vi "FRIC_navX_Internal_I2C_ProcessingLoop.vi"(10 "I2C Bus (in)":T3=enum."Invalid", 11 "Update Rate (4Hz-100Hz)":u8=50 min=4 max=100) -> (0 "error out":errorcluster)   [LabVIEW 2015]
doc: "This navX VI handles the reading/writing for the navX. All of the good stuff is in here.\nTHIS VI SHOULD NOT BE CALLED BY THE USER!"
uses:
  <vilib>/Rock Robotics/SystemInterfaces/i2clib/i2c_bus.ctl
  navX Library v2/_TypeDefs/Z900_navX_DeviceTypeDef.ctl
  navX Library v2/_TypeDefs/Z900_navX_ProtocolTypeDef.ctl
  navX Library v2/_TypeDefs/Z900_navX_NotifyPacketTypeDef.ctl
  navX Library v2/_TypeDefs/Z900_navX_ActionTypeDef.ctl
  TypeDefs/FRIC_navX_ProcessingLoopStatesTypeDef_I2C.ctl
  TypeDefs/FRIC_navX_I2C Process Loop TypeDef.ctl
  <vilib>/Rock Robotics/SystemInterfaces/Typedef/FPGA_TypedefDigitalModule.ctl
  navX Library v2/_TypeDefs/Z900_navX_IntegrationControlRegisters.ctl
  <vilib>/Rock Robotics/WPI/SPI/WPI_SPIDevRef.ctl
  <vilib>/Rock Robotics/SystemInterfaces/spilib/spi_bus.ctl
  _NI WPI Serial USB/WPI_SerialPort_USB.ctl
  navX Library v2/_TypeDefs/Z900_navX_SerialStreamTypeDef.ctl
  <vilib>/Rock Robotics/WPI/SerialPort/WPI_SerialPortRef.ctl
  navX Library v2/_TypeDefs/Flags/Z900_navX_Flags_CapabilityTypeDef.ctl
  navX Library v2/_TypeDefs/Z900_navX_DeviceRegisters.ctl
  navX Library v2/_TypeDefs/navX Open TypeDefs/Z900_navX_OpenTypeDef_I2C.ctl
  <vilib>/Rock Robotics/SystemInterfaces/Utilities/FPGA_UtilitiesRead LocalTime.vi
  navX Library v2/navX Library v2.lvlib
  _NI WPI Serial USB/_NI WPI Serial USB.lvlib
panel:
  out "output cluster":T1={"Interface"={"Protocol"=enum."SERIAL", "Update Rate (4Hz-100Hz)"=4, "navX Open TypeDef"=variant}, "Notify Packet"=refnum, "Loop VI Refnum"=refnum, "Ready to Close Occurrence Refnum"=refnum, "Name"=""} {"Interface"."Update Rate (4Hz-100Hz)" min=4 max=60 step=1}
  out "Connected":bool
  in  "Halt":bool
  out "Registry":u8[](array[numeric])
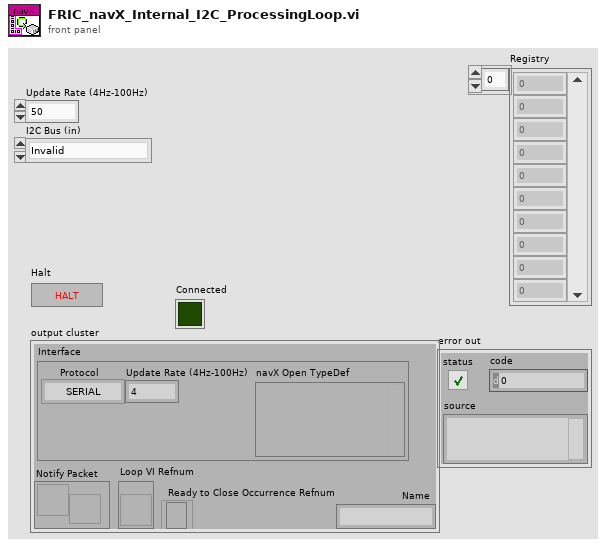
[diagram p1: front panel]
types:
  T1 = typedef "navX Library v2.lvlib/Z900_navX_DeviceTypeDef.ctl" = cluster{"Interface":cluster{"Protocol":T2, "Update Rate (4Hz-100Hz)":u8, "navX Open TypeDef":variant}, "Notify Packet":refnum<notifier>, "Loop VI Refnum":refnum<vi>, "Ready to Close Occurrence Refnum":refnum<k4>, "Name":string}
  T2 = typedef "navX Library v2.lvlib/Z900_navX_ProtocolTypeDef.ctl" = enum16{"SERIAL", "I2C", "SPI"}
  T3 = typedef "i2c_bus.ctl" = enum16{"I2C On-Board", "I2C MXP", "Invalid"}
  T4 = typedef "FRIC_navX_ProcessingLoopStatesTypeDef_I2C.ctl" = enum16{"Process", "INI", "Check Packets Valid", "Close", "Decode Serial Packet", "Flush Serial", "Generate Command", "Last Packet Valid", "Open", "Read", "Reset Serial", "Set Termination Char", "Wait", "Write", "Exit"}
  T5 = typedef "FRIC_navX_I2C Process Loop TypeDef.ctl" = cluster{"State Array":T4[], "error":errorcluster, "FPGA Cluster":cluster{"Last Valid FPGA Time":dbl, "Error Count":i32, "Initialized":bool}, "Device Info":T1, "I2CDevRef":cluster{"DevStatus":errorcluster, "Controller":T6, "Device Address":u8, "Handle":i32, "I2C Bus":T3}, "Registry":u8[], "Command Array":T7[], "Connected?":bool, "navX Device Memory Size":i32, "notification":T8, "Memory Size Set":bool, "SPIDevRef":T10, "navX Serial Open":cluster{"Serial Port":T12, "Stream Type":T13}, "SerialPortRef":T14, "Serial Read Buffer":string, "Serial Write Buffer":string[]}
  T6 = typedef "FPGA_TypedefDigitalModule.ctl" = enum16{"Controller 1"}
  T7 = typedef "navX Library v2.lvlib/Z900_navX_IntegrationControlRegisters.ctl" = u8
  T8 = typedef "navX Library v2.lvlib/Z900_navX_NotifyPacketTypeDef.ctl" = cluster{"navX Action":T9, "Data":variant}
  T9 = typedef "navX Library v2.lvlib/Z900_navX_ActionTypeDef.ctl" = enum16{"None", "Halt", "Normal Read", "Update Serial Protocol", "Update Rate Htz", "Zero-Yaw", "Zero-Displacement", "Zero-Velocity"}
  T10 = typedef "WPI_SPIDevRef.ctl" = cluster{"DevStatus":errorcluster, "Handle":i32, "Controller":T6, "SPI Bus":T11}
  T11 = typedef "spi_bus.ctl" = enum16{"SPI On-Board, CS0", "SPI On-Board, CS1", "SPI On-Board, CS2", "SPI On-Board, CS3", "SPI MXP", "Invalid"}
  T12 = typedef "_NI WPI Serial USB.lvlib/WPI_SerialPort_USB.ctl" = enum16{"Onboard RS-232", "MXP TTL", "USB"}
  T13 = typedef "navX Library v2.lvlib/Z900_navX_SerialStreamTypeDef.ctl" = enum16{"YRPH", "Quaterinons", "Gyro/Raw", "AHRS", "AHRSAndPositioning"}
  T14 = typedef "WPI_SerialPortRef.ctl" = cluster{"DevStatus":errorcluster, "Serial Port Name":refnum<visa-resource-name>}
  T15 = typedef "navX Library v2.lvlib/Z900_navX_OpenTypeDef_I2C.ctl" = cluster{"I2C Bus":T3}
  T16 = typedef "navX Library v2.lvlib/Z900_navX_DeviceRegisters.ctl" = u8
  T17 = typedef "navX Library v2.lvlib/Z900_navX_Flags_CapabilityTypeDef.ctl" = u16
  T18 = cluster{"DevStatus":errorcluster, "Controller":T6, "Device Address":u8, "Handle":i32, "I2C Bus":T3}
  T19 = cluster{"Last Valid FPGA Time":dbl, "Error Count":i32, "Initialized":bool}
  T20 = typedef "WPI_I2CDevRef.ctl" = cluster{"DevStatus":errorcluster, "Controller":T6, "Device Address":u8, "Handle":i32, "I2C Bus":T3}
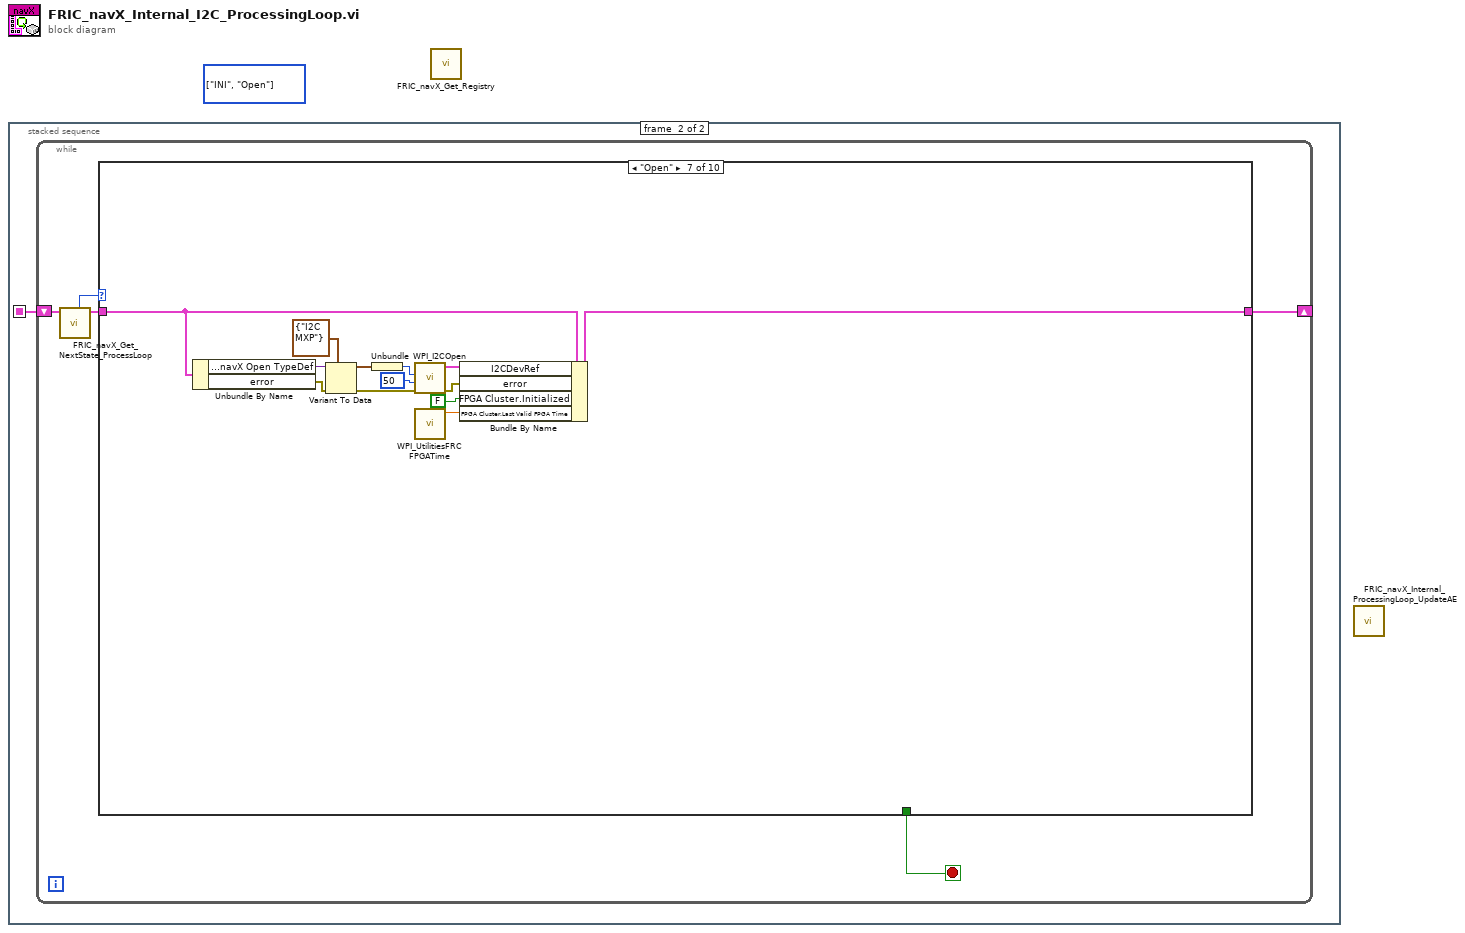
[diagram p0: block diagram]
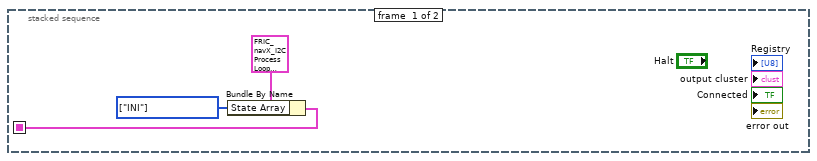
[diagram p2: hidden frame]
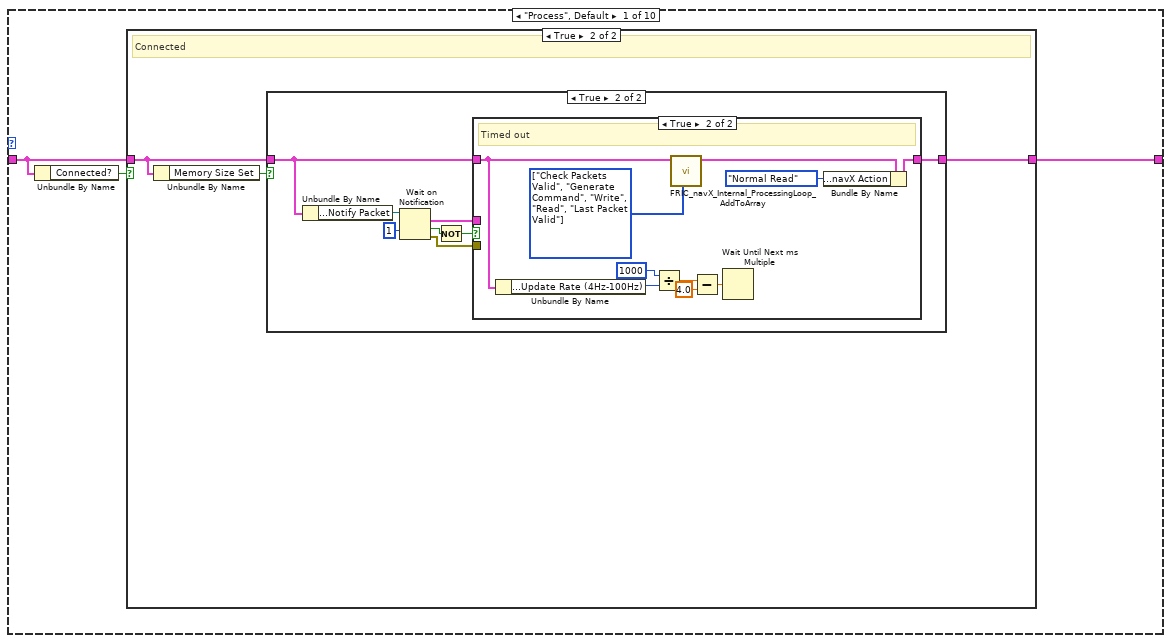
[diagram p3: hidden frame]
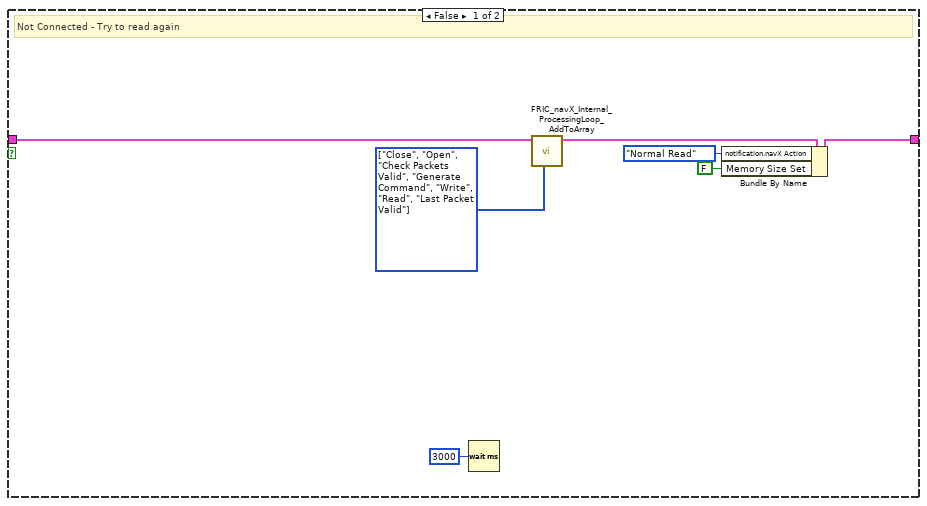
[diagram p4: hidden frame]
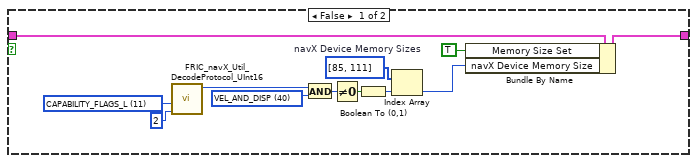
[diagram p5: hidden frame]
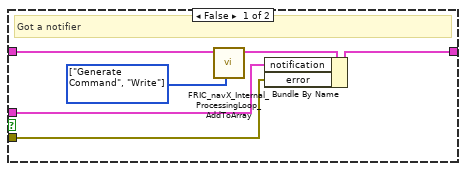
[diagram p6: hidden frame]
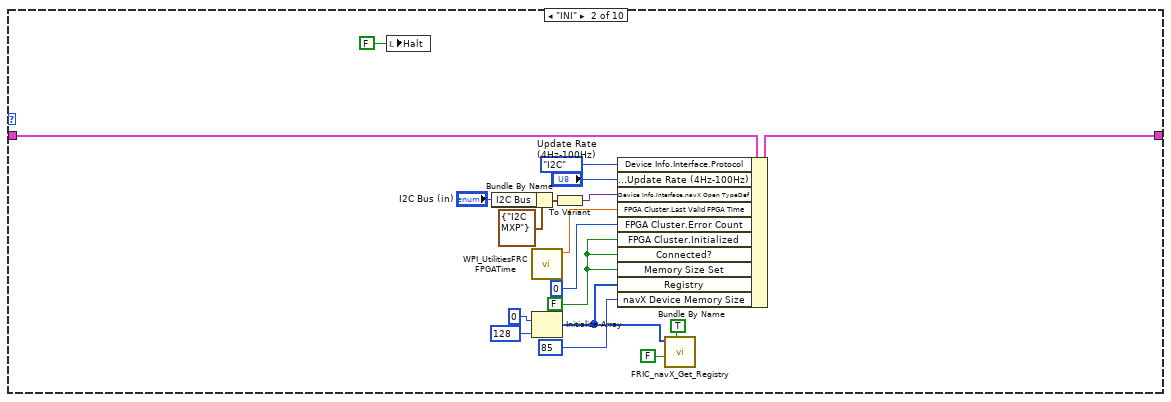
[diagram p7: hidden frame]
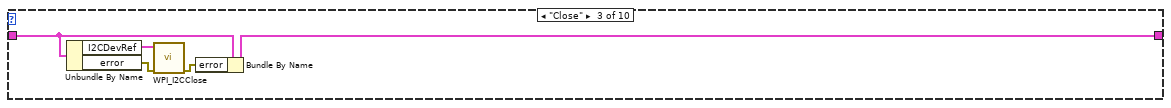
[diagram p8: hidden frame]
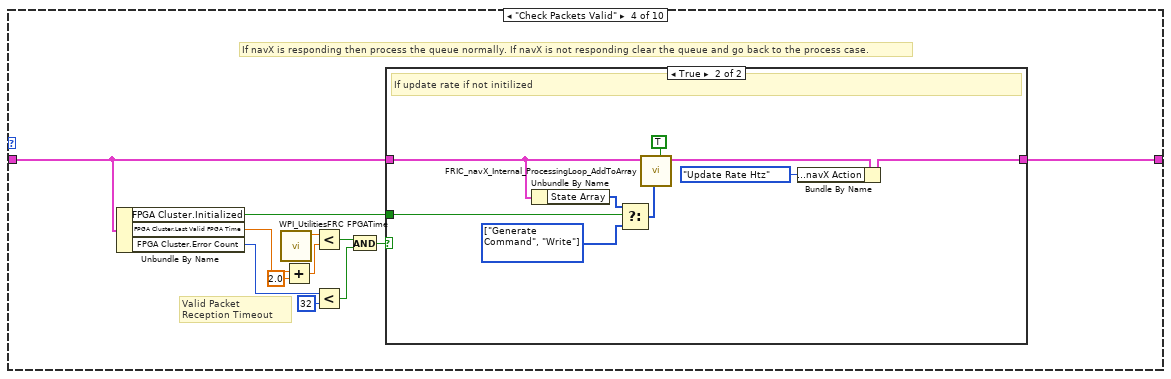
[diagram p9: hidden frame]
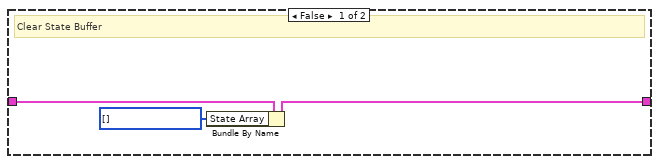
[diagram p10: hidden frame]
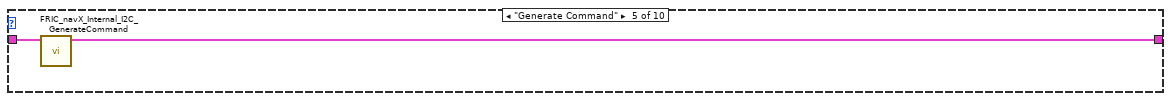
[diagram p11: hidden frame]
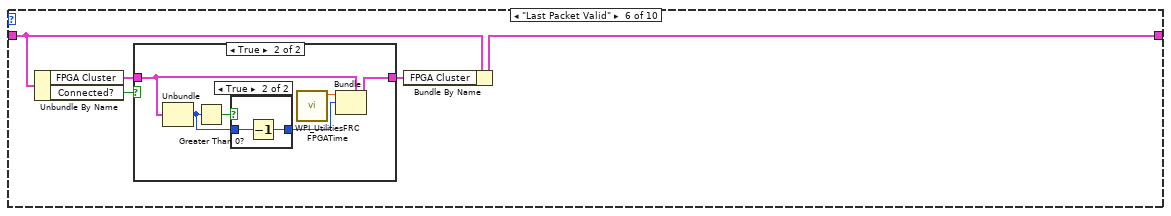
[diagram p12: hidden frame]
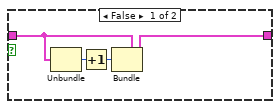
[diagram p13: hidden frame]
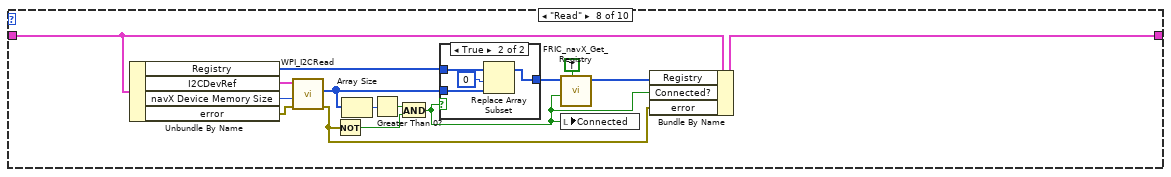
[diagram p15: hidden frame]
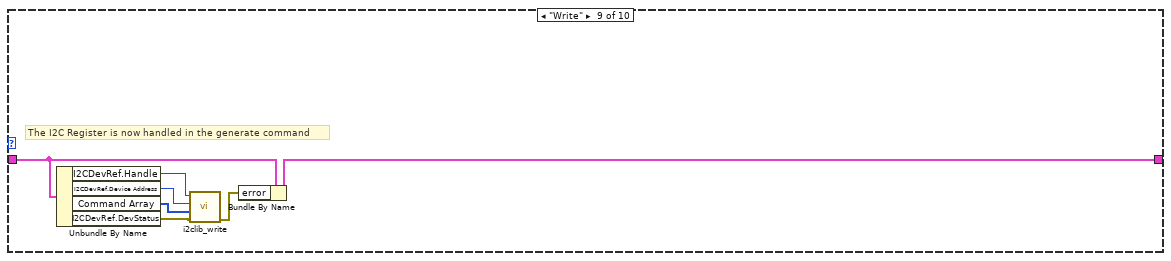
[diagram p17: hidden frame]
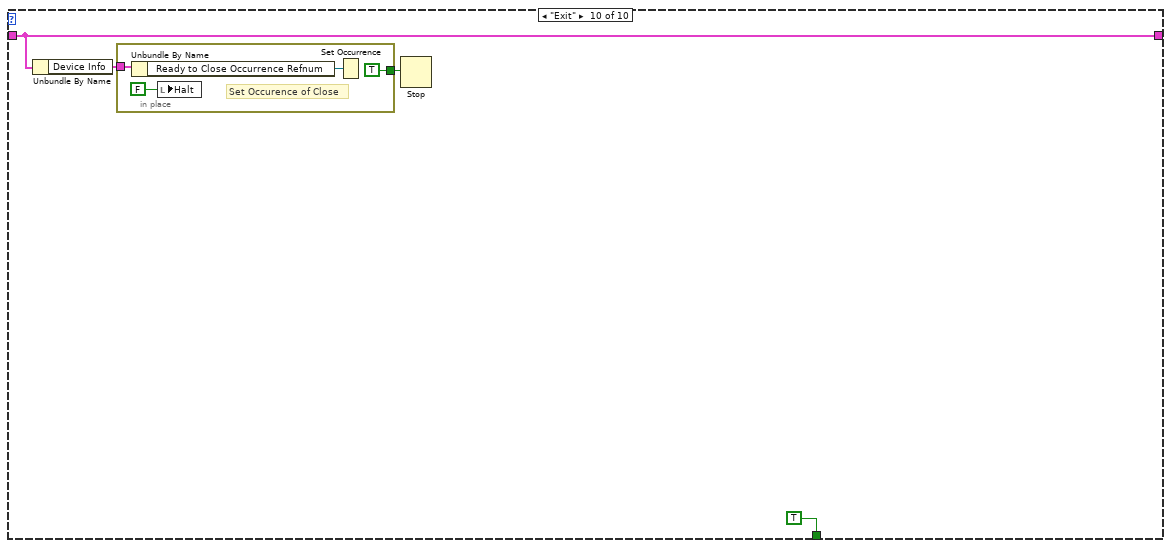
[diagram p18: hidden frame]
diagram:
  (unwired) T4[] [enum."INI", enum."Open"] items=["Process", "INI", "Check Packets Valid", "Close", "Decode Serial Packet", "Flush Serial", "Generate Command", "Last Packet Valid", "Open", "Read", "Reset Serial", "Set Termination Char", "Wait", "Write", "Exit"]
  n1 = stacked-sequence {
    seq-local: [w3 _] -> [_ w4]
    frame #0 {
      w1 = T4[] [enum."INI"] items=["Process", "INI", "Check Packets Valid", "Close", "Decode Serial Packet", "Flush Serial", "Generate Command", "Last Packet Valid", "Open", "Read", "Reset Serial", "Set Termination Char", "Wait", "Write", "Exit"] ("State Array")
      n2 = Bundle By Name(cluster=T5 {"State Array"=[enum."INI", enum."Open"], "error"={"status"=FALSE, "code"=0, "source"=""}, "FPGA Cluster"={"Last Valid FPGA Time"=0.0, "Error Count"=0, "Initialized"=FALSE}, "Device Info"={"Interface"={"Protocol"=enum."SERIAL", "Update Rate (4Hz-100Hz)"=4, "navX Open TypeDef"=variant}, "Notify Packet"=refnum, "Loop VI Refnum"=refnum, "Ready to Close Occurrence Refnum"=refnum, "Name"=""}, "I2CDevRef"={"DevStatus"={"status"=FALSE, "code"=0, "source"=""}, "Controller"=enum."Controller 1", "Device Address"=0, "Handle"=0, "I2C Bus"=enum."Invalid"}, "Registry"=[], "Command Array"=[214, 32], "Connected?"=FALSE, "navX Device Memory Size"=85, "notification"={"navX Action"=enum."None", "Data"=variant}, "Memory Size Set"=FALSE, "SPIDevRef"={"DevStatus"={"status"=FALSE, "code"=0, "source"=""}, "Handle"=0, "Controller"=enum."Controller 1", "SPI Bus"=enum."SPI On-Board, CS0"}, "navX Serial Open"={"Serial Port"=enum."Onboard RS-232", "Stream Type"=enum."YRPH"}, "SerialPortRef"={"DevStatus"={"status"=FALSE, "code"=0, "source"=""}, "Serial Port Name"=""}, "Serial Read Buffer"="", "Serial Write Buffer"=[]} ("I2C Process Loop TypeDef"), "State Array"=w1) -> (w3:T5)
    }
    frame #1 {
      n3 = while {
        shift-right: [w5] -> _
        shift-left: w4 -> [w8]
        stop <- w9 stop-if-true
        n4 = call "FRIC_navX_Get_NextState_ProcessLoop.vi"("I2C Process Loop TypeDef (in)"=w8) -> ("I2C Process Loop TypeDef (out)"=w7:T5, "Current State"=w6:T4)  [unwired: 9 in]
        n5 = case shown="\"Open\"" w6 {
          tunnel: [_ _ _ _ _ _ _ _ _ TRUE] -> w9
          tunnel: w7 -> [w10 w70 w79 w85 w107 w111 w131 w144 w164 w167]
          tunnel: [w12 w64 w78 w86 w106 w110 w130 w143 w165 w167] -> w5
          frame "Process", Default {
            n6 = Unbundle By Name(w10) -> ("Connected?"=w11:bool)
            n7 = case shown="True" w11 {
              tunnel: w10 -> [w18 w21]
              tunnel: [w15 w22] -> w12
              frame False {
                w17 = T4[] [enum."Close", enum."Open", enum."Check Packets Valid", enum."Generate Command", enum."Write", enum."Read", enum."Last Packet Valid"] items=["Process", "INI", "Check Packets Valid", "Close", "Decode Serial Packet", "Flush Serial", "Generate Command", "Last Packet Valid", "Open", "Read", "Reset Serial", "Set Termination Char", "Wait", "Write", "Exit"]
                # "Not Connected - Try to read again"
                n8 = Wait (ms)(milliseconds to wait=u32 3000) -> ()  [unwired: 1 out]
                n9 = call "FRIC_navX_Internal_ProcessingLoop_AddToArray.vi"("States Array"=w17, "I2C Process Loop TypeDef (in)"=w18) -> ("I2C Process Loop TypeDef (out)"=w16:T5)  [unwired: 9 in]
                n10 = Bundle By Name(cluster=w16, "notification.navX Action"=Z900_navX_ActionTypeDef."Normal Read", "Memory Size Set"=FALSE) -> (w15:T5)
              }
              frame True {
                # "Connected"
                n11 = Unbundle By Name(w21) -> ("Memory Size Set"=w20:bool)
                n12 = case shown="True" w20 {
                  tunnel: [w33 w39] -> w22
                  tunnel: w21 -> [w34 w35]
                  frame False {
                    w32 = T16 11 items=["WHOAMI"=0, "HW_REV"=1, "FW_VER_MAJOR"=2, "FW_VER_MINOR"=3, "UPDATE_RATE_HZ"=4, "ACCEL_FSR_G"=5, "GYRO_FSR_DPS"=6, "OP_STATUS"=8, "CAL_STATUS"=9, "SELFTEST_STATUS"=10, "CAPABILITY_FLAGS_L"=11, "CAPABILITY_FLAGS_H"=12, "SENSOR_STATUS"=16, "TIMESTAMP"=18, "YAW"=22, "ROLL"=24, "PITCH"=26, "HEADING"=28, "FUSED_HEADING"=30, "ALTITUDE_I"=32, "ALTITUDE_D"=34, "LINERA_ACC_X"=36, "LINERA_ACC_Y"=38, "LINERA_ACC_Z"=40, "QUAT_W"=42, "QUAT_X"=44, "QUAT_Y"=46, "QUAT_Z"=48, "MPU_TEMP_C"=50, "GYRO_X"=52, "GYRO_Y"=54, "GYRO_Z"=56, "ACC_X"=58, "ACC_Y"=60, "ACC_Z"=62, "MAG_X"=64, "MAG_Y"=66, "MAG_Z"=68, "PRESSURE_I"=70, "PRESSURE_D"=72, "PRESSURE_TEMP"=74, "YAW_OFFSET"=76, "QUAT_OFFSET_W"=78, "QUAT_OFFSET_X"=80, "QUAT_OFFSET_Y"=82, "QUAT_OFFSET_Z"=84, "INTEGRATION_CONTROL"=86, "VELOCITY_X"=88, "VELOCITY_Y"=92, "VELOCITY_Z"=96, "DISPLACMENT_X"=100, "DISPLACMENT_Y"=104, "DISPLACEMENT_Z"=108] ("Device Register")
                    w27 = T17 40 items=["OMNIMOUNT"=4, "OMNIMOUNT_CONFIG_MASK"=38, "VEL_AND_DISP"=40, "YAW_RESET"=80] ("Capability Flag")
                    w28 = i32[] [85, 111]  # navX Device Memory Sizes
                    n13 = call "FRIC_navX_Util_DecodeProtocol_UInt16.vi"("length"=2, "Device Register"=w32) -> ("Value"=w25:u16)  [unwired: 9 in]
                    n14 = And(x=w25, y=w27) -> (x .and. y?=w26:T17)
                    n15 = Not Equal To 0?(x=w26) -> (x != 0?=w29:bool)
                    n16 = Boolean To (0,1)(Boolean=w29) -> (0, 1=w30:i16)
                    n17 = Index Array(array=w28, index=w30) -> (element=w24:i32)
                    n18 = Bundle By Name(cluster=w34, "Memory Size Set"=TRUE, "navX Device Memory Size"=w24) -> (w33:T5)
                  }
                  frame True {
                    n19 = Unbundle By Name(w35) -> ("Device Info.Notify Packet"=w42:refnum<notifier>)
                    n20 = Wait on Notification(notifier=w42, timeout in ms (-1)=1) -> (notification=w37:T8, timed out?=w40:bool, error out=w36:errorcluster)  [unwired: 2 in, 1 out]
                    n21 = Not(x=w40) -> (.not. x?=w38:bool)
                    n22 = case shown="True" w38 {
                      tunnel: w35 -> [w48 w52]
                      tunnel: [w47 w50] -> w39
                      tunnel: w37 -> [w46 _]
                      tunnel: w36 -> [w43 _]
                      frame False {
                        w44 = T4[] [enum."Generate Command", enum."Write"] items=["Process", "INI", "Check Packets Valid", "Close", "Decode Serial Packet", "Flush Serial", "Generate Command", "Last Packet Valid", "Open", "Read", "Reset Serial", "Set Termination Char", "Wait", "Write", "Exit"] ("States Array")
                        # "Got a notifier"
                        n23 = call "FRIC_navX_Internal_ProcessingLoop_AddToArray.vi"("States Array"=w44, "I2C Process Loop TypeDef (in)"=w48) -> ("I2C Process Loop TypeDef (out)"=w45:T5)  [unwired: 9 in]
                        n24 = Bundle By Name(cluster=w45, "notification"=w46, "error"=w43) -> (w47:T5)
                      }
                      frame True {
                        w53 = T4[] [enum."Check Packets Valid", enum."Generate Command", enum."Write", enum."Read", enum."Last Packet Valid"] items=["Process", "INI", "Check Packets Valid", "Close", "Decode Serial Packet", "Flush Serial", "Generate Command", "Last Packet Valid", "Open", "Read", "Reset Serial", "Set Termination Char", "Wait", "Write", "Exit"]
                        # "Timed out"
                        n25 = Unbundle By Name(w52) -> ("Device Info.Interface.Update Rate (4Hz-100Hz)"=w58:u8)
                        n26 = Divide(x=i16 1000, y=w58) -> (x/y=w56:dbl)
                        n27 = call "FRIC_navX_Internal_ProcessingLoop_AddToArray.vi"("States Array"=w53, "I2C Process Loop TypeDef (in)"=w52) -> ("I2C Process Loop TypeDef (out)"=w51:T5)  [unwired: 9 in]
                        n28 = Subtract(x=w56, y=4.0) -> (x-y=w54:dbl)
                        n29 = Wait Until Next ms Multiple(millisecond multiple=w54) -> ()  [unwired: 1 out]
                        n30 = Bundle By Name(cluster=w51, "notification.navX Action"=Z900_navX_ActionTypeDef."Normal Read") -> (w50:T5)
                      }
                    }
                  }
                }
              }
            }
          }
          frame "INI" {
            w62 = FALSE ("Initialized")
            n31 = local write "Halt"(FALSE ("Halt")) -> ()
            n32 = Bundle By Name(cluster=T15 {"I2C Bus"=enum."I2C MXP"} ("navX I2C Open"), "I2C Bus"="I2C Bus (in)") -> (w71:T15)
            n33 = call <vilib>:"WPI_UtilitiesFRC FPGATime.vi"() -> ("FPGA Time"=w66:dbl)  [unwired: 10 in, 1 out]
            n34 = Initialize Array(u8 0 ("Received Data"), 128 ("hex")) -> (w59:u8[])
            n35 = To Variant(anything=w71) -> (Variant=w67:variant)
            n36 = Bundle By Name(cluster=w70, "Device Info.Interface.Protocol"=Z900_navX_ProtocolTypeDef."I2C" ("Protocol"), "Device Info.Interface.Update Rate (4Hz-100Hz)"="Update Rate (4Hz-100Hz)", "Device Info.Interface.navX Open TypeDef"=w67, "FPGA Cluster.Last Valid FPGA Time"=w66, "FPGA Cluster.Error Count"=0 ("Error Count"), "FPGA Cluster.Initialized"=w62, "Connected?"=w62, "Memory Size Set"=w62, "Registry"=w59, "navX Device Memory Size"=85 ("hex")) -> (w64:T5)
            n37 = call "FRIC_navX_Get_Registry.vi"("Update"=TRUE, "Connected?"=FALSE, "Registry (in)"=w59) -> ()  [unwired: 7 in, 2 out]
          }
          frame "Close" {
            n38 = Unbundle By Name(w79) -> ("I2CDevRef"=w81:T18, "error"=w80:errorcluster)
            n39 = call <vilib>:"WPI_I2CClose.vi"("error in (no error)"=w80, "I2CDevRef"=w81) -> ("error out"=w77:errorcluster)  [unwired: 9 in]
            n40 = Bundle By Name(cluster=w79, "error"=w77) -> (w78:T5)
          }
          frame "Check Packets Valid" {
            # "If navX is responding then process the queue normally. If navX is not responding clear the queue and go back to the process case."
            # "Valid Packet Reception Timeout"
            n41 = Unbundle By Name(w85) -> ("FPGA Cluster.Initialized"=w83:bool, "FPGA Cluster.Last Valid FPGA Time"=w84:dbl, "FPGA Cluster.Error Count"=w82:i32)
            n42 = call <vilib>:"WPI_UtilitiesFRC FPGATime.vi"() -> ("FPGA Time"=w91:dbl)  [unwired: 10 in, 1 out]
            n43 = Add(x=w84, y=2.0) -> (x+y=w92:dbl)
            n44 = Less?(x=w91, y=w92) -> (x < y?=w89:bool)
            n45 = Less?(x=w82, y=32) -> (x < y?=w88:bool)
            n46 = And(x=w89, y=w88) -> (x .and. y?=w87:bool)
            n47 = case shown="True" w87 {
              tunnel: w85 -> [w96 w103]
              tunnel: [w95 w98] -> w86
              tunnel: w83 -> [_ w104]
              frame False {
                w94 = T4[] [] items=["Process", "INI", "Check Packets Valid", "Close", "Decode Serial Packet", "Flush Serial", "Generate Command", "Last Packet Valid", "Open", "Read", "Reset Serial", "Set Termination Char", "Wait", "Write", "Exit"] ("f")
                # "Clear State Buffer"
                n48 = Bundle By Name(cluster=w96, "State Array"=w94) -> (w95:T5)
              }
              frame True {
                w100 = T4[] [enum."Generate Command", enum."Write"] items=["Process", "INI", "Check Packets Valid", "Close", "Decode Serial Packet", "Flush Serial", "Generate Command", "Last Packet Valid", "Open", "Read", "Reset Serial", "Set Termination Char", "Wait", "Write", "Exit"] ("f")
                # "If update rate if not initilized"
                n49 = Unbundle By Name(w103) -> ("State Array"=w102:T4[])
                n50 = Select(t=w102, s=w104, f=w100) -> (s? t:f=w101:T4[])
                n51 = call "FRIC_navX_Internal_ProcessingLoop_AddToArray.vi"("Add to beginning"=TRUE, "States Array"=w101, "I2C Process Loop TypeDef (in)"=w103) -> ("I2C Process Loop TypeDef (out)"=w99:T5)  [unwired: 8 in]
                n52 = Bundle By Name(cluster=w99, "notification.navX Action"=Z900_navX_ActionTypeDef."Update Rate Htz") -> (w98:T5)
              }
            }
          }
          frame "Generate Command" {
            n53 = call "FRIC_navX_Internal_I2C_GenerateCommand.vi"("I2C Process Loop TypeDef (in)"=w107) -> ("I2C Process Loop TypeDef (out)"=w106:T5)  [unwired: 10 in]
          }
          frame "Last Packet Valid" {
            n54 = Unbundle By Name(w111) -> ("FPGA Cluster"=w112:T19, "Connected?"=w108:bool)
            n55 = case shown="True" w108 {
              tunnel: [w115 w122] -> w109
              tunnel: w112 -> [w114 w118]
              frame False {
                n56 = Unbundle(w114) -> ("Error Count"=w113:i32)  [unwired: 2 out]
                n57 = Increment(x=w113) -> (x+1=w116:i32)
                n58 = Bundle(cluster=w114, "Error Count"=w116) -> (w115:T19)  [unwired: 2 in]
              }
              frame True {
                n59 = Unbundle(w118) -> ("Error Count"=w117:i32)  [unwired: 2 out]
                n60 = Greater Than 0?(x=w117) -> (x > 0?=w120:bool)
                n61 = case shown="True" w120 {
                  tunnel: [w123 w125] -> w119
                  tunnel: w117 -> [w123 w124]
                  frame False {
                  }
                  frame True {
                    n62 = Decrement(x=w124) -> (x-1=w125:i32)
                  }
                }
                n63 = call <vilib>:"WPI_UtilitiesFRC FPGATime.vi"() -> ("FPGA Time"=w121:dbl)  [unwired: 10 in, 1 out]
                n64 = Bundle(cluster=w118, "Last Valid FPGA Time"=w121, "Error Count"=w119) -> (w122:T19)  [unwired: 1 in]
              }
            }
            n65 = Bundle By Name(cluster=w111, "FPGA Cluster"=w109) -> (w110:T5)
          }
          frame "Open" {
            n66 = Unbundle By Name(w131) -> ("Device Info.Interface.navX Open TypeDef"=w138:variant, "error"=w128:errorcluster)
            n67 = Variant To Data(error in=w128, type=T15 {"I2C Bus"=enum."I2C MXP"} ("navX I2C Open"), Variant=w138) -> (data=w137:T15, error out=w133:errorcluster)
            n68 = Unbundle(w137) -> ("I2C Bus"=w135:T3)
            n69 = call <vilib>:"WPI_I2COpen.vi"("error in"=w133, "Device Address"=u8 50, "I2C Bus"=w135) -> ("error out"=w129:errorcluster, "I2CDevRef"=w132:T20)  [unwired: 7 in]
            n70 = call <vilib>:"WPI_UtilitiesFRC FPGATime.vi"() -> ("FPGA Time"=w126:dbl)  [unwired: 10 in, 1 out]
            n71 = Bundle By Name(cluster=w131, "I2CDevRef"=w132, "error"=w129, "FPGA Cluster.Initialized"=FALSE ("Initialized"), "FPGA Cluster.Last Valid FPGA Time"=w126) -> (w130:T5)
          }
          frame "Read" {
            n72 = Unbundle By Name(w144) -> ("Registry"=w139:u8[], "I2CDevRef"=w147:T18, "navX Device Memory Size"=w145:i32, "error"=w146:errorcluster)
            n73 = call <vilib>:"WPI_I2CRead.vi"("error in (no error)"=w146, "I2CBytesToRead"=w145, "I2CDevRef"=w147) -> ("error out"=w140:errorcluster, "Data Out"=w151:u8[])  [unwired: 6 in, 1 out]
            n74 = Not(x=w140) -> (.not. x?=w148:bool)
            n75 = Array Size(array=w151) -> (size(s)=w150:i32)
            n76 = Greater Than 0?(x=w150) -> (x > 0?=w149:bool)
            n77 = And(x=w149, y=w148) -> (x .and. y?=w141:bool)
            n78 = case shown="True" w141 {
              tunnel: w139 -> [w154 w158]
              tunnel: [w154 w157] -> w153
              tunnel: w151 -> [_ w156]
              frame False {
              }
              frame True {
                n79 = Replace Array Subset(array=w158, new element=w156, index=u8 0 ("hex")) -> (w157:u8[])
              }
            }
            n80 = call "FRIC_navX_Get_Registry.vi"("Update"=TRUE, "Connected?"=w141, "Registry (in)"=w153) -> ("Registry (out)"=w142:u8[])  [unwired: 7 in, 1 out]
            n81 = local write "Connected"(w141) -> ()
            n82 = Bundle By Name(cluster=w144, "Registry"=w142, "Connected?"=w141, "error"=w140) -> (w143:T5)
          }
          frame "Write" {
            # "The I2C Register is now handled in the generate command"
            n83 = Unbundle By Name(w164) -> ("I2CDevRef.Handle"=w163:i32, "I2CDevRef.Device Address"=w162:u8, "Command Array"=w160:T7[], "I2CDevRef.DevStatus"=w161:errorcluster)
            n84 = call <vilib>:"i2clib_write.vi"("error in (no error)"=w161, "send_data"=w160, "dev_addr"=w162, "I2C Reference"=w163) -> ("error out"=w159:errorcluster)  [unwired: 6 in, 1 out]
            n85 = Bundle By Name(cluster=w164, "error"=w159) -> (w165:T5)
          }
          frame "Exit" {
            n86 = Unbundle By Name(w167) -> ("Device Info"=w166:T1)
            n87 = in-place {
              in-place-border: w166 -> [w170]
              in-place-border: [TRUE] -> w169
              # "Set Occurence of Close"
              n88 = Unbundle By Name(w170) -> ("Ready to Close Occurrence Refnum"=w172:refnum<k4>)
              n89 = local write "Halt"(FALSE ("Halt")) -> ()
              n90 = Set Occurrence(w172) -> ()
            }
            n91 = Stop(stop? (T)=w169) -> ()
          }
        }
      }
    }
  }
  n92 = call "FRIC_navX_Get_Registry.vi"() -> ()  [unwired: 10 in, 2 out]
  n93 = call "FRIC_navX_Internal_ProcessingLoop_UpdateAE.vi"() -> ()  [unwired: 6 in, 10 out]
